vi "testCreateTCPIPConnectionServersAandB.vi"(8 "error in":errorcluster) -> (0 "error out":errorcluster)   [LabVIEW 2018]
doc: "This test shows that runServer.vi for servers A and B cannot run and stop at same time."
uses:
  <vilib>/addons/_JKI Toolkits/Caraya/classes/Assert/Assert Not Error.vi
  src/TcpServer/TcpServer.lvclass
  <vilib>/addons/_JKI Toolkits/Caraya/classes/Test/Test.lvclass
  <vilib>/addons/_JKI Toolkits/Caraya/classes/Assert/Assert.lvclass
panel:
  out "Run Server B error out":errorcluster
  out "Run Server A error out":errorcluster
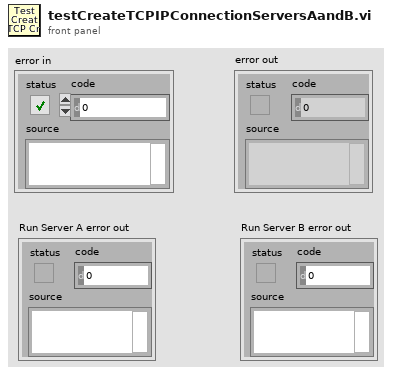
[diagram p1: front panel]
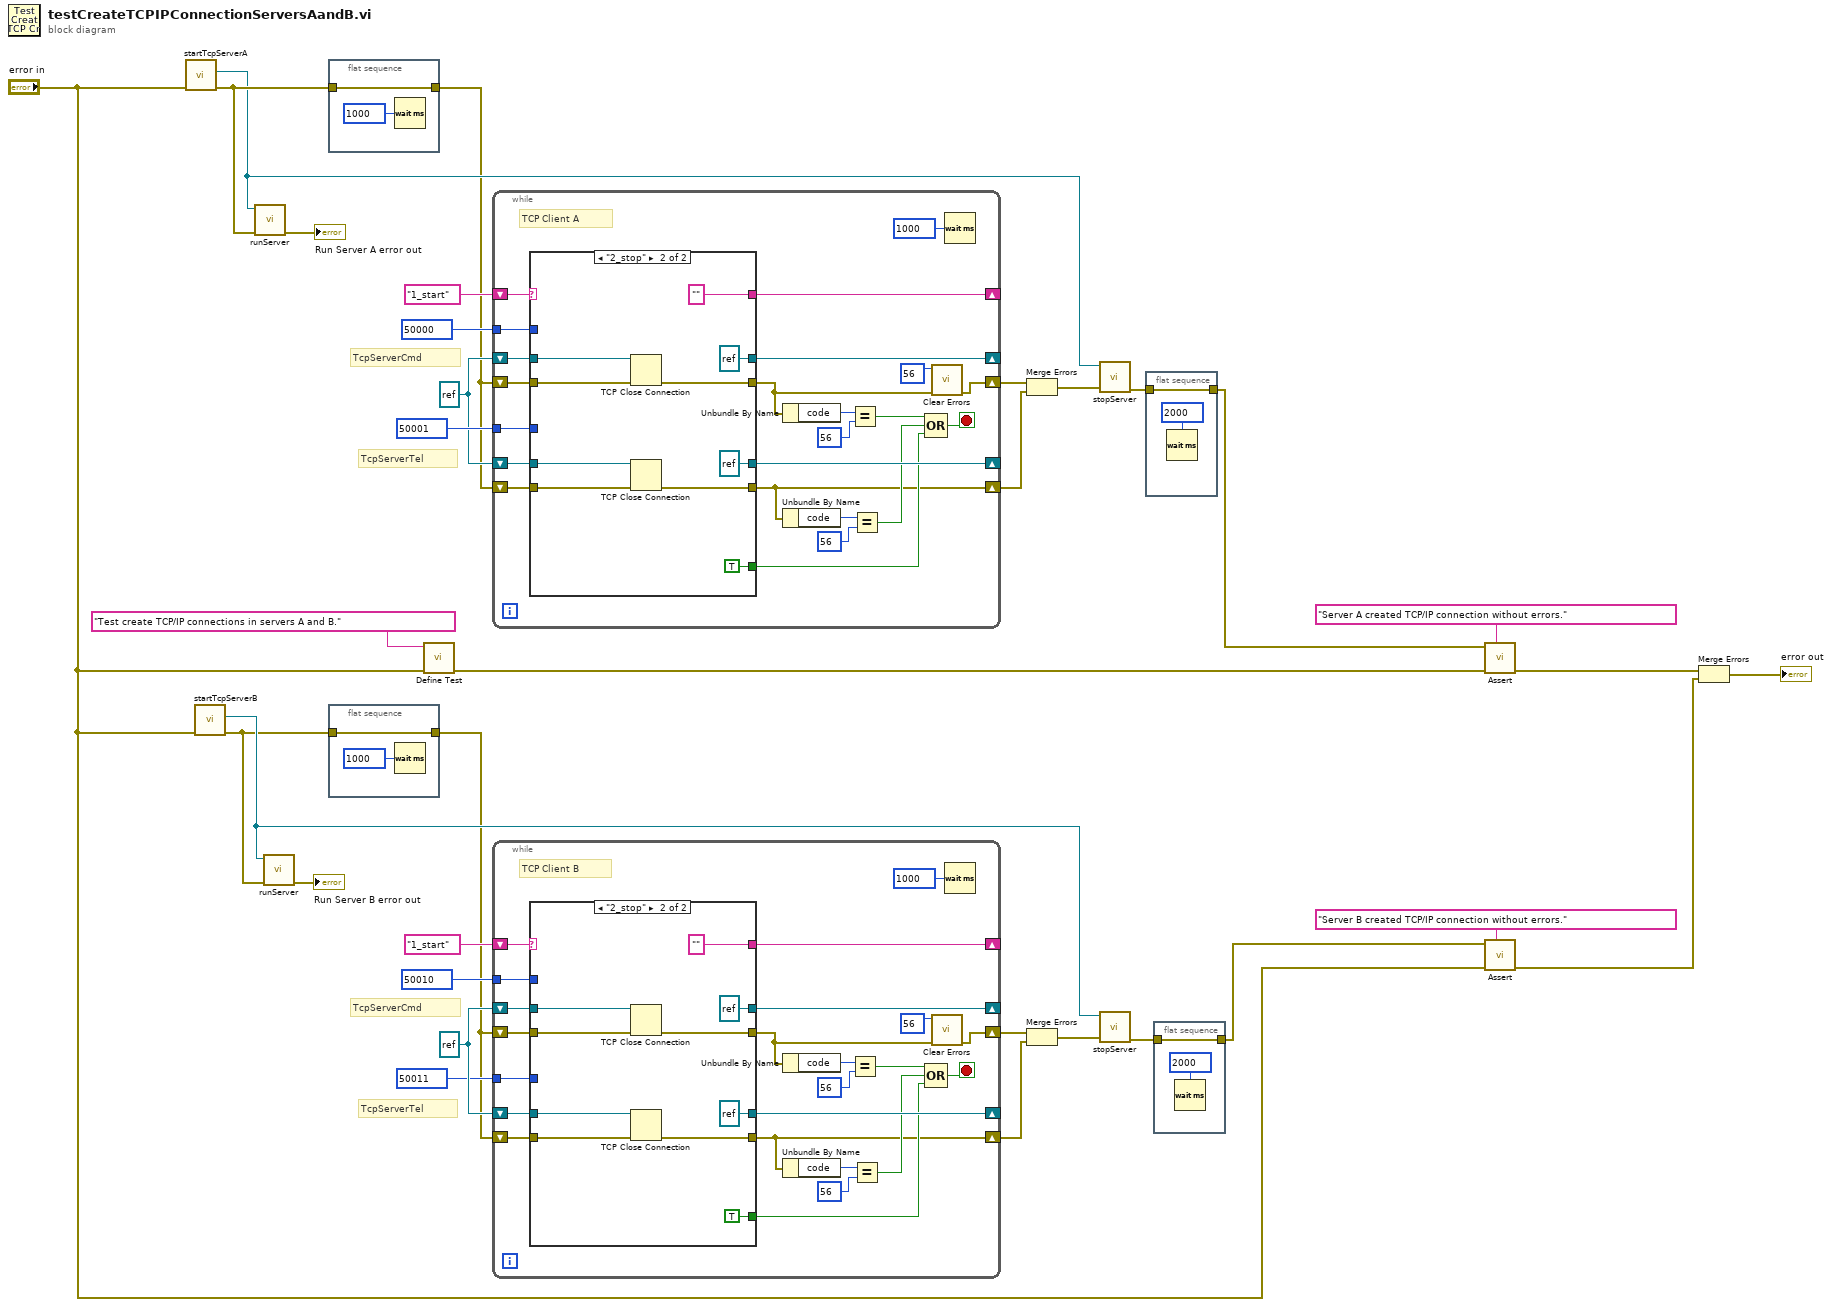
[diagram p0: block diagram]
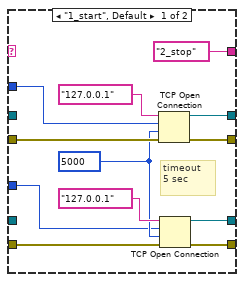
[diagram p2: hidden frame]
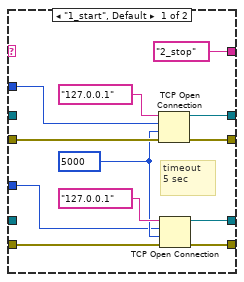
[diagram p3: hidden frame]
diagram:
  w20 = refnum<k5> refnum ("connection ID")
  w22 = refnum<k5> refnum ("connection ID")
  # "TcpServerTel"
  # "TcpServerCmd"
  # "TcpServerTel"
  # "TcpServerCmd"
  n1 = call "startTcpServerA.vi"("error in (no error)"="error in") -> ("error out"=w23:errorcluster, "TcpServer out"=w21:refnum<class "TcpServer.lvclass">)  [unwired: 8 in, 1 out]
  n2 = call "startTcpServerB.vi"("error in (no error)"="error in") -> ("error out"=w2:errorcluster, "TcpServer out"=w13:refnum<class "TcpServer.lvclass">)  [unwired: 8 in, 1 out]
  n3 = call "runServer.vi"("error in (no error)"=w23, "TcpServer in"=w21) -> ("error out (no error)"=→"Run Server A error out":errorcluster)  [unwired: 8 in, 1 out]
  n4 = call "runServer.vi"("error in (no error)"=w2, "TcpServer in"=w13) -> ("error out (no error)"=→"Run Server B error out":errorcluster)  [unwired: 8 in, 1 out]
  n5 = flat-sequence {
    tunnel: w23 -> [w35]
    tunnel: [w35] -> w3
    frame #0 {
      n6 = Wait (ms)(milliseconds to wait=u32 1000) -> ()  [unwired: 1 out]
    }
  }
  n7 = flat-sequence {
    tunnel: w2 -> [w37]
    tunnel: [w37] -> w12
    frame #0 {
      n8 = Wait (ms)(milliseconds to wait=u32 1000) -> ()  [unwired: 1 out]
    }
  }
  n9 = call <vilib>:"Define Test.vi"("error in (no error)"="error in", "Label (VI Title)"="Test create TCP/IP connections in servers A and B.") -> ("error out"=w25:errorcluster)  [unwired: 9 in]
  n10 = while {
    shift-right: [w54] -> _
    shift-left: "1_start" ("address") -> [w61]
    shift-right: [w60] -> _
    shift-left: w22 -> [w58]
    shift-right: [w59] -> _
    shift-left: w22 -> [w57]
    shift-right: [w47] -> w30
    shift-left: w3 -> [w56]
    shift-right: [w42] -> w31
    shift-left: w3 -> [w55]
    tunnel: u16 50000 ("remote port or service name") -> [w40]
    tunnel: u16 50001 ("remote port or service name") -> [w39]
    stop <- w48 stop-if-true
    # "TCP Client A"
    n11 = case shown="\"2_stop\"" w61 {
      tunnel: [w71 refnum<k5> refnum ("connection ID")] -> w60
      tunnel: [w70 refnum<k5> refnum ("connection ID")] -> w59
      tunnel: w58 -> [_ w83]
      tunnel: w57 -> [_ w81]
      tunnel: [w69 w79] -> w44
      tunnel: [w68 w78] -> w42
      tunnel: w56 -> [w66 w82]
      tunnel: w55 -> [w65 w80]
      tunnel: ["2_stop" ("address") "" ("address")] -> w54
      tunnel: [_ TRUE] -> w45
      tunnel: w40 -> [w63 _]
      tunnel: w39 -> [w62 _]
      frame "1_start", Default {
        w64 = 5000 ("timeout ms (60000)")
        # "timeout\n5 sec"
        n12 = TCP Open Connection(address="127.0.0.1", remote port or service name=w63, timeout ms (60000)=w64, error in (no error)=w66) -> (connection ID=w71:refnum<k5>, error out=w69:errorcluster)  [unwired: 1 in]
        n13 = TCP Open Connection(address="127.0.0.1", remote port or service name=w62, timeout ms (60000)=w64, error in (no error)=w65) -> (connection ID=w70:refnum<k5>, error out=w68:errorcluster)  [unwired: 1 in]
      }
      frame "2_stop" {
        n14 = TCP Close Connection(connection ID=w83, error in (no error)=w82) -> (error out=w79:errorcluster)  [unwired: 1 in, 1 out]
        n15 = TCP Close Connection(connection ID=w81, error in (no error)=w80) -> (error out=w78:errorcluster)  [unwired: 1 in, 1 out]
      }
    }
    n16 = Unbundle By Name(w44) -> ("code"=w43:i32)
    n17 = Unbundle By Name(w42) -> ("code"=w41:i32)
    n18 = Equal?(x=w43, y=56) -> (x = y?=w50:bool)
    n19 = Equal?(x=w41, y=56) -> (x = y?=w49:bool)
    n20 = Compound Arithmetic op=OR(w50, w49, w45) -> (w48:bool)
    n21 = call <vilib>:"Clear Errors.vi"("error in (no error)"=w44, "specific error code to clear (0: all)"=56) -> ("error out"=w47:errorcluster)  [unwired: 4 in, 1 out]
    n22 = Wait (ms)(milliseconds to wait=u32 1000) -> ()  [unwired: 1 out]
  }
  n23 = while {
    shift-right: [w99] -> _
    shift-left: "1_start" ("address") -> [w106]
    shift-right: [w105] -> _
    shift-left: w20 -> [w103]
    shift-right: [w104] -> _
    shift-left: w20 -> [w102]
    shift-right: [w92] -> w17
    shift-left: w12 -> [w101]
    shift-right: [w87] -> w16
    shift-left: w12 -> [w100]
    tunnel: u16 50010 ("remote port or service name") -> [w85]
    tunnel: u16 50011 ("remote port or service name") -> [w84]
    stop <- w93 stop-if-true
    # "TCP Client B"
    n24 = case shown="\"2_stop\"" w106 {
      tunnel: [w116 refnum<k5> refnum ("connection ID")] -> w105
      tunnel: [w115 refnum<k5> refnum ("connection ID")] -> w104
      tunnel: w103 -> [_ w128]
      tunnel: w102 -> [_ w126]
      tunnel: [w114 w124] -> w89
      tunnel: [w113 w123] -> w87
      tunnel: w101 -> [w111 w127]
      tunnel: w100 -> [w110 w125]
      tunnel: ["2_stop" ("address") "" ("address")] -> w99
      tunnel: [_ TRUE] -> w90
      tunnel: w85 -> [w108 _]
      tunnel: w84 -> [w107 _]
      frame "1_start", Default {
        w109 = 5000 ("timeout ms (60000)")
        # "timeout\n5 sec"
        n25 = TCP Open Connection(address="127.0.0.1", remote port or service name=w108, timeout ms (60000)=w109, error in (no error)=w111) -> (connection ID=w116:refnum<k5>, error out=w114:errorcluster)  [unwired: 1 in]
        n26 = TCP Open Connection(address="127.0.0.1", remote port or service name=w107, timeout ms (60000)=w109, error in (no error)=w110) -> (connection ID=w115:refnum<k5>, error out=w113:errorcluster)  [unwired: 1 in]
      }
      frame "2_stop" {
        n27 = TCP Close Connection(connection ID=w128, error in (no error)=w127) -> (error out=w124:errorcluster)  [unwired: 1 in, 1 out]
        n28 = TCP Close Connection(connection ID=w126, error in (no error)=w125) -> (error out=w123:errorcluster)  [unwired: 1 in, 1 out]
      }
    }
    n29 = Unbundle By Name(w89) -> ("code"=w88:i32)
    n30 = Unbundle By Name(w87) -> ("code"=w86:i32)
    n31 = Equal?(x=w88, y=56) -> (x = y?=w95:bool)
    n32 = Equal?(x=w86, y=56) -> (x = y?=w94:bool)
    n33 = Compound Arithmetic op=OR(w95, w94, w90) -> (w93:bool)
    n34 = call <vilib>:"Clear Errors.vi"("error in (no error)"=w89, "specific error code to clear (0: all)"=56) -> ("error out"=w92:errorcluster)  [unwired: 4 in, 1 out]
    n35 = Wait (ms)(milliseconds to wait=u32 1000) -> ()  [unwired: 1 out]
  }
  n36 = Merge Errors(w30, w31) -> (w29:errorcluster)
  n37 = Merge Errors(w17, w16) -> (w18:errorcluster)
  n38 = call "stopServer.vi"("error in (no error)"=w29, "tcpServer in"=w21) -> ("error out"=w26:errorcluster)  [unwired: 8 in, 1 out]
  n39 = call "stopServer.vi"("error in (no error)"=w18, "tcpServer in"=w13) -> ("error out"=w11:errorcluster)  [unwired: 8 in, 1 out]
  n40 = flat-sequence {
    tunnel: w26 -> [w129]
    tunnel: [w129] -> w10
    frame #0 {
      n41 = Wait (ms)(milliseconds to wait=u32 2000) -> ()  [unwired: 1 out]
    }
  }
  n42 = flat-sequence {
    tunnel: w11 -> [w131]
    tunnel: [w131] -> w6
    frame #0 {
      n43 = Wait (ms)(milliseconds to wait=u32 2000) -> ()  [unwired: 1 out]
    }
  }
  n44 = call-poly <vilib>:"Assert.vi"("Label"="Server A created TCP/IP connection without errors.", "error in (no error)"=w25, "Not Error?"=w10) -> ("error out"=w24:errorcluster)  [unwired: 8 in]
  n45 = call-poly <vilib>:"Assert.vi"("Label"="Server B created TCP/IP connection without errors.", "error in (no error)"="error in", "Not Error?"=w6) -> ("error out"=w4:errorcluster)  [unwired: 8 in]
  n46 = Merge Errors(w24, w4) -> (→"error out":errorcluster)
